vi "Test Tokenizer Absolute Single Command Formats.vi"(8 "error in (no error)":errorcluster) -> (0 "error out":errorcluster)   [LabVIEW 2019]
uses:
  PathTokenizer/PathTokenizer.lvclass
  PathTokenizer/PathTokenizer.lvclass/PathTokenizer.ctl
  <vilib>/addons/_JKI Toolkits/Caraya/classes/Assert/Assert Equal Value_Variant.vi
  <vilib>/addons/_JKI Toolkits/Caraya/classes/Assert/Assert.lvclass
  <vilib>/addons/_JKI Toolkits/Caraya/classes/Test/Test.lvclass
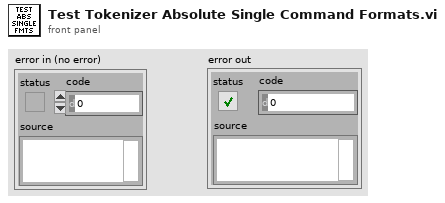
[diagram p1: front panel]
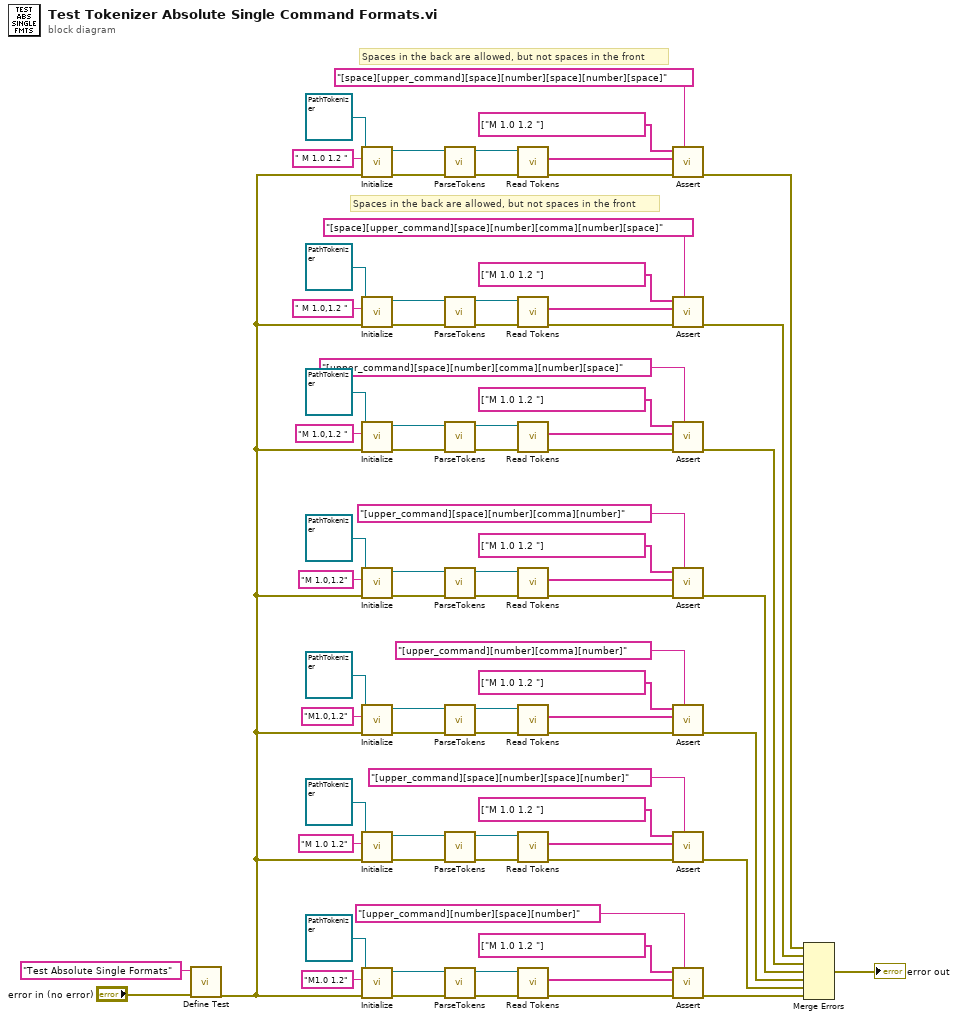
[diagram p0: block diagram]
diagram:
  # "Spaces in the back are allowed, but not spaces in the front"
  # "Spaces in the back are allowed, but not spaces in the front"
  n1 = call <vilib>:"Define Test.vi"("error in (no error)"="error in (no error)", "Label (VI Title)"="Test Absolute Single Formats") -> ("error out"=w3:errorcluster)  [unwired: 8 in, 1 out]
  n2 = call "Initialize.vi"("error in (no error)"=w3, "Path Command Text"=" M 1.0 1.2 ", "PathTokenizer in"=refnum<class "PathTokenizer.lvclass"> refnum) -> ("error out"=w19:errorcluster, "PathTokenizer out"=w18:refnum<class "PathTokenizer.lvclass">)  [unwired: 7 in]
  n3 = call "Initialize.vi"("error in (no error)"=w3, "Path Command Text"=" M 1.0,1.2 ", "PathTokenizer in"=refnum<class "PathTokenizer.lvclass"> refnum) -> ("error out"=w20:errorcluster, "PathTokenizer out"=w21:refnum<class "PathTokenizer.lvclass">)  [unwired: 7 in]
  n4 = call "Initialize.vi"("error in (no error)"=w3, "Path Command Text"="M 1.0,1.2 ", "PathTokenizer in"=refnum<class "PathTokenizer.lvclass"> refnum) -> ("error out"=w39:errorcluster, "PathTokenizer out"=w38:refnum<class "PathTokenizer.lvclass">)  [unwired: 7 in]
  n5 = call "Initialize.vi"("error in (no error)"=w3, "Path Command Text"="M 1.0,1.2", "PathTokenizer in"=refnum<class "PathTokenizer.lvclass"> refnum) -> ("error out"=w40:errorcluster, "PathTokenizer out"=w41:refnum<class "PathTokenizer.lvclass">)  [unwired: 7 in]
  n6 = call "Initialize.vi"("error in (no error)"=w3, "Path Command Text"="M1.0,1.2", "PathTokenizer in"=refnum<class "PathTokenizer.lvclass"> refnum) -> ("error out"=w59:errorcluster, "PathTokenizer out"=w58:refnum<class "PathTokenizer.lvclass">)  [unwired: 7 in]
  n7 = call "Initialize.vi"("error in (no error)"=w3, "Path Command Text"="M 1.0 1.2", "PathTokenizer in"=refnum<class "PathTokenizer.lvclass"> refnum) -> ("error out"=w60:errorcluster, "PathTokenizer out"=w61:refnum<class "PathTokenizer.lvclass">)  [unwired: 7 in]
  n8 = call "Initialize.vi"("error in (no error)"=w3, "Path Command Text"="M1.0 1.2", "PathTokenizer in"=refnum<class "PathTokenizer.lvclass"> refnum) -> ("error out"=w80:errorcluster, "PathTokenizer out"=w79:refnum<class "PathTokenizer.lvclass">)  [unwired: 7 in]
  n9 = call "ParseTokens.vi"("error in (no error)"=w19, "PathTokenizer in"=w18) -> ("error out"=w14:errorcluster, "PathTokenizer out"=w15:refnum<class "PathTokenizer.lvclass">)  [unwired: 8 in]
  n10 = call "ParseTokens.vi"("error in (no error)"=w20, "PathTokenizer in"=w21) -> ("error out"=w25:errorcluster, "PathTokenizer out"=w24:refnum<class "PathTokenizer.lvclass">)  [unwired: 8 in]
  n11 = call "ParseTokens.vi"("error in (no error)"=w39, "PathTokenizer in"=w38) -> ("error out"=w34:errorcluster, "PathTokenizer out"=w35:refnum<class "PathTokenizer.lvclass">)  [unwired: 8 in]
  n12 = call "ParseTokens.vi"("error in (no error)"=w40, "PathTokenizer in"=w41) -> ("error out"=w45:errorcluster, "PathTokenizer out"=w44:refnum<class "PathTokenizer.lvclass">)  [unwired: 8 in]
  n13 = call "ParseTokens.vi"("error in (no error)"=w59, "PathTokenizer in"=w58) -> ("error out"=w54:errorcluster, "PathTokenizer out"=w55:refnum<class "PathTokenizer.lvclass">)  [unwired: 8 in]
  n14 = call "ParseTokens.vi"("error in (no error)"=w60, "PathTokenizer in"=w61) -> ("error out"=w65:errorcluster, "PathTokenizer out"=w64:refnum<class "PathTokenizer.lvclass">)  [unwired: 8 in]
  n15 = call "ParseTokens.vi"("error in (no error)"=w80, "PathTokenizer in"=w79) -> ("error out"=w75:errorcluster, "PathTokenizer out"=w76:refnum<class "PathTokenizer.lvclass">)  [unwired: 8 in]
  n16 = call "Read Tokens.vi"("error in (no error)"=w14, "PathTokenizer in"=w15) -> ("error out"=w11:errorcluster, "Tokens"=w13:string[])  [unwired: 7 in, 1 out]
  n17 = call "Read Tokens.vi"("error in (no error)"=w25, "PathTokenizer in"=w24) -> ("error out"=w28:errorcluster, "Tokens"=w26:string[])  [unwired: 7 in, 1 out]
  n18 = call "Read Tokens.vi"("error in (no error)"=w34, "PathTokenizer in"=w35) -> ("error out"=w31:errorcluster, "Tokens"=w33:string[])  [unwired: 7 in, 1 out]
  n19 = call "Read Tokens.vi"("error in (no error)"=w45, "PathTokenizer in"=w44) -> ("error out"=w48:errorcluster, "Tokens"=w46:string[])  [unwired: 7 in, 1 out]
  n20 = call "Read Tokens.vi"("error in (no error)"=w54, "PathTokenizer in"=w55) -> ("error out"=w51:errorcluster, "Tokens"=w53:string[])  [unwired: 7 in, 1 out]
  n21 = call "Read Tokens.vi"("error in (no error)"=w65, "PathTokenizer in"=w64) -> ("error out"=w68:errorcluster, "Tokens"=w66:string[])  [unwired: 7 in, 1 out]
  n22 = call "Read Tokens.vi"("error in (no error)"=w75, "PathTokenizer in"=w76) -> ("error out"=w72:errorcluster, "Tokens"=w74:string[])  [unwired: 7 in, 1 out]
  n23 = call-poly <vilib>:"Assert.vi"("Label"="[space][upper_command][space][number][space][number][space]", "error in (no error)"=w11, "Y"=w13, "X"=string[] ["M 1.0 1.2 "] ("Tokens")) -> ("error out"=w4:errorcluster)  [unwired: 6 in, 1 out]
  n24 = call-poly <vilib>:"Assert.vi"("Label"="[space][upper_command][space][number][comma][number][space]", "error in (no error)"=w28, "Y"=w26, "X"=string[] ["M 1.0 1.2 "] ("Tokens")) -> ("error out"=w5:errorcluster)  [unwired: 6 in, 1 out]
  n25 = call-poly <vilib>:"Assert.vi"("Label"="[upper_command][space][number][comma][number][space]", "error in (no error)"=w31, "Y"=w33, "X"=string[] ["M 1.0 1.2 "] ("Tokens")) -> ("error out"=w6:errorcluster)  [unwired: 6 in, 1 out]
  n26 = call-poly <vilib>:"Assert.vi"("Label"="[upper_command][space][number][comma][number]", "error in (no error)"=w48, "Y"=w46, "X"=string[] ["M 1.0 1.2 "] ("Tokens")) -> ("error out"=w7:errorcluster)  [unwired: 6 in, 1 out]
  n27 = call-poly <vilib>:"Assert.vi"("Label"="[upper_command][number][comma][number]", "error in (no error)"=w51, "Y"=w53, "X"=string[] ["M 1.0 1.2 "] ("Tokens")) -> ("error out"=w8:errorcluster)  [unwired: 6 in, 1 out]
  n28 = call-poly <vilib>:"Assert.vi"("Label"="[upper_command][space][number][space][number]", "error in (no error)"=w68, "Y"=w66, "X"=string[] ["M 1.0 1.2 "] ("Tokens")) -> ("error out"=w9:errorcluster)  [unwired: 6 in, 1 out]
  n29 = call-poly <vilib>:"Assert.vi"("Label"="[upper_command][number][space][number]", "error in (no error)"=w72, "Y"=w74, "X"=string[] ["M 1.0 1.2 "] ("Tokens")) -> ("error out"=w70:errorcluster)  [unwired: 6 in, 1 out]
  n30 = Merge Errors(w4, w5, w6, w7, w8, w9, w70) -> (→"error out":errorcluster)
